vi "Get Index of Single Wheel from Name.vi"(8 "error in (no error)":errorcluster, 10 "wheel name":string, 11 "steering frame in":refnum<class "NI_Robotics_Steering Frame.lvclass">) -> (0 "error out":errorcluster, 1 "found?":bool, 2 "index":i32, 3 "steering frame out":refnum<class "NI_Robotics_Steering Frame.lvclass">)   [LabVIEW 2017, in "NI_Robotics_Steering Frame.lvclass"]
uses:
  <vilib>/robotics/Steering/Steering Frame/NI_Robotics_Steering Frame.lvclass
  <vilib>/robotics/Steering/Steering Frame/NI_Robotics_Steering Frame.lvclass/NI_Robotics_Steering Frame.ctl
  <vilib>/robotics/Steering/Wheel/NI_Robotics_Wheel.lvclass/NI_Robotics_Wheel.ctl
  <vilib>/robotics/Steering/Wheel/Get Wheel Name.vi
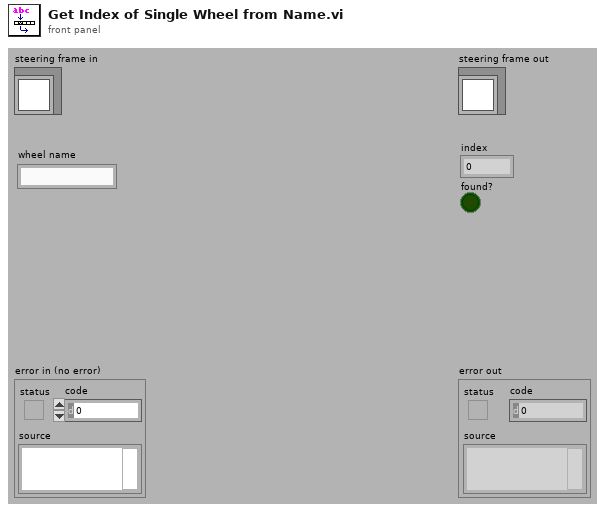
[diagram p1: front panel]
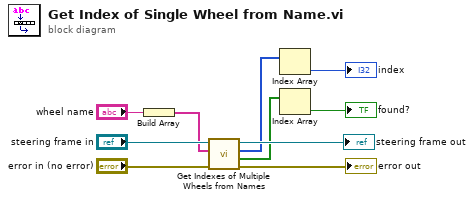
[diagram p0: block diagram]
diagram:
  n1 = Build Array("wheel name") -> (w8:string[])
  n2 = call <vilib>:"Get Indexes of Multiple Wheels from Names.vi"("error in (no error)"="error in (no error)", "wheel names"=w8, "steering frame in"="steering frame in") -> ("error out"=→"error out":errorcluster, "found?"=w2:bool[], "indexes"=w4:i32[], "steering frame out"=→"steering frame out":refnum<class "NI_Robotics_Steering Frame.lvclass">)  [unwired: 5 in]
  n3 = Index Array(array=w4) -> (element=→"index":i32)  [unwired: 1 in]
  n4 = Index Array(array=w2) -> (element=→"found?":bool)  [unwired: 1 in]
